vi "Init DAQ Analog Out.vi"(8 "error in":errorcluster, 10 "name to assign":string, 11 "physical channels":tag) -> (0 "error out":errorcluster, 3 "Refnum out":refnum<k21>)   [LabVIEW 2021]
uses:
  <vilib>/DAQmx/create/channels.llb/DAQmx Create Channel (AO-Voltage-Basic).vi
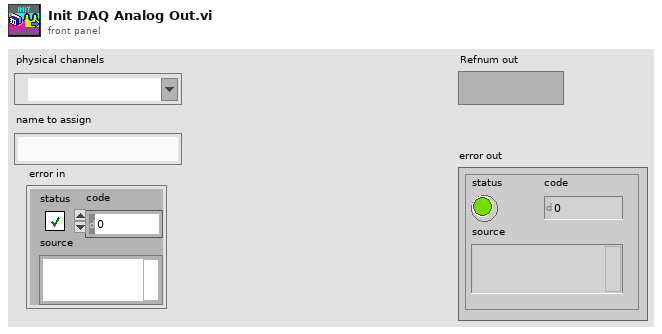
[diagram p1: front panel]
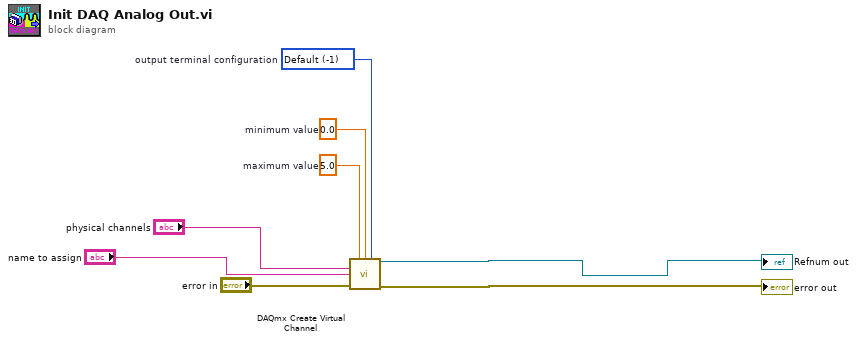
[diagram p0: block diagram]
diagram:
  w3 = -1 items=["Default"=-1, "RSE"=10083, "Differential"=10106, "Pseudodifferential"=12529]  # output terminal configuration
  w4 = 5.0  # maximum value
  w5 = 0.0  # minimum value
  n1 = call-poly <vilib>:"DAQmx Create Virtual Channel.vi"("maximum value"=w4, "minimum value"=w5, "output terminal configuration"=w3, "physical channels"="physical channels", "name to assign"="name to assign", "error in"="error in") -> ("task out"=→"Refnum out":refnum<k21>, "error out"=→"error out":errorcluster)  [unwired: 8 in]
